vi "Mutex Create Object.vi"(8 "error in (no error)":errorcluster, 11 "mutex pointer in":u64) -> (0 "error out":errorcluster, 3 "Mutex out":T1)   [LabVIEW 2013, in "Linux RT IPC.lvlib" / "POSIX Threads.lvlib" / "Mutex.lvclass"]
doc: "Creates a LabVIEW object used to encapsulate a pthread mutex object referenced by mutex pointer."
uses:
  Mutex.lvclass
  Controls/reference.ctl
  POSIX Thread Object/POSIX Thread Object.lvclass/POSIX Thread Object.ctl
  POSIX Thread Object/POSIX Thread Object.lvclass
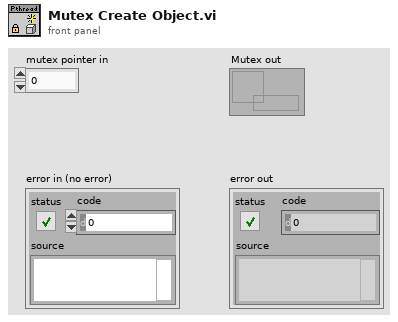
[diagram p1: front panel]
types:
  T1 = typedef "Linux RT IPC.lvlib/POSIX Threads.lvlib/Mutex.lvclass/reference.ctl" = refnum<data-value>
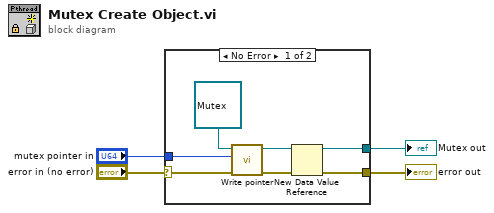
[diagram p0: block diagram]
diagram:
  n1 = case shown="No Error" "error in (no error)" {
    selector: "error in (no error)" -> [w7 w12]
    tunnel: "mutex pointer in" -> [w8 _]
    tunnel: [w6 w12] -> w2
    tunnel: [w5 _] -> w1
    frame No Error {
      n2 = call "Write pointer.vi"("error in (no error)"=w7, "pointer"=w8, "POSIX Thread Object in"=refnum<class "Mutex.lvclass"> refnum ("POSIX Threads.lvlib:Mutex.lvclass")) -> ("error out"=w9:errorcluster, "POSIX Thread Object out"=w10:refnum<class "Mutex.lvclass">)  [unwired: 7 in]
      n3 = New Data Value Reference(data value=w10, error in=w9) -> (data value reference=w5:refnum<data-value>, error out=w6:errorcluster)
    }
    frame Error {
    }
  }
  "Mutex out" <- w1
  "error out" <- w2
